vi "Get-file-names.vi"(8 "error in (no error)":errorcluster, 11 "Object ref in":T1) -> (0 "error out":errorcluster, 2 "Files list":string[][](array[string]), 3 "Object ref out":T1)   [LabVIEW 2013, in "SLMControl.lvlib" / "SC-Main.lvclass"]
uses:
  SC-Main.lvclass
  Object-reference.ctl
  UI/Control-names.ctl
  SC-Main.lvclass/SC-Main.ctl
  Read UI.vi
  Read Lasing files.vi
  Read Deposition files.vi
  UI/SC-UI.lvclass
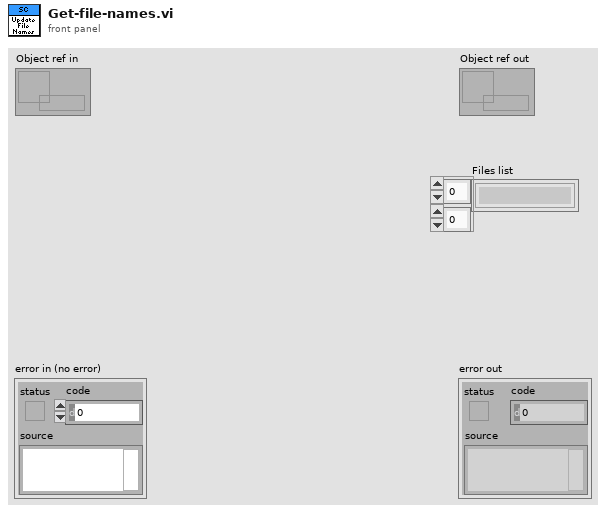
[diagram p1: front panel]
types:
  T1 = typedef "SLMControl.lvlib/SC-Main.lvclass/Object-reference.ctl" = refnum<data-value>
  T2 = typedef "SLMControl.lvlib/SC-UI.lvclass/Control-names.ctl" = enum16{"Com-in", "Com-out", "Help", "Status", "Load configuration", "Save configuration", "Load lasing files", "Load deposition files", "Clear", "Files", "Activate", "Execute", "Abort", "Options", "Current layer", "Current iteration", "Last elapsed time", "Deposition status", "Lasing job", "Status LEDs", "Exiting led", "Initialized led", "Files loaded led", "Activated led", "Executing led", "Deposition led", "Lasing job led", "Lasing led"}
  T3 = typedef "SLMControl.lvlib/SC-UI.lvclass/Panes-reference.ctl" = refnum<data-value>
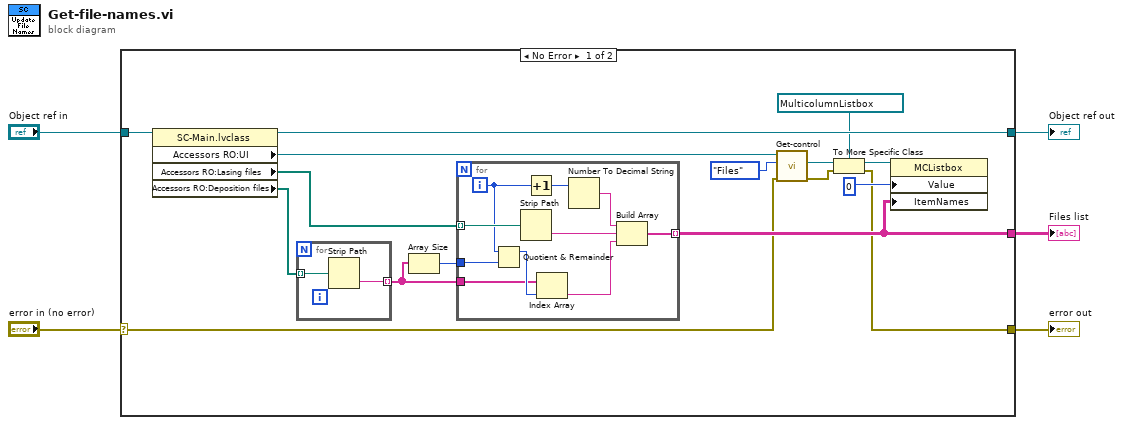
[diagram p0: block diagram]
diagram:
  n1 = case shown="No Error" "error in (no error)" {
    selector: "error in (no error)" -> [w8 w35]
    tunnel: [w6 w35] -> w4
    tunnel: [w20 w34] -> w2
    tunnel: "Object ref in" -> [w21 w34]
    tunnel: [w10 _] -> w1
    frame No Error {
      n2 = property class="SC-Main.lvclass"(reference=w21) -> (reference out=w20:T1, "Accessors RO:UI"=w15:T3, "Accessors RO:Lasing files"=w16:path[], "Accessors RO:Deposition files"=w19:path[])  [unwired: 1 in, 1 out]
      n3 = for {
        tunnel: w19 -> [w23] mode=indexing
        tunnel: [w22] -> w17 mode=indexing
        n4 = Strip Path(path=w23) -> (name=w22:string)  [unwired: 1 out]
      }
      n5 = Array Size(array=w17) -> (size(s)=w18:i32)
      n6 = for {
        tunnel: w16 -> [w33] mode=indexing
        tunnel: [w24] -> w10 mode=indexing
        tunnel: w17 -> [w26]
        tunnel: w18 -> [w29]
        i -> [w28]
        n7 = Quotient & Remainder(x=w28, y=w29) -> (x-y*floor(x/y)=w27:i32)  [unwired: 1 out]
        n8 = Strip Path(path=w33) -> (name=w30:string)  [unwired: 1 out]
        n9 = Increment(x=w28) -> (x+1=w32:i32)
        n10 = Index Array(array=w26, index=w27) -> (element=w25:string)
        n11 = Number To Decimal String(number=w32) -> (decimal integer string=w31:string)  [unwired: 1 in]
        n12 = Build Array(w31, w30, w25) -> (w24:string[])
      }
      n13 = call "Get-control.vi"("error in (no error)"=w8, "Control name"=Control-names."Files", "Panes in"=w15) -> ("error out"=w7:errorcluster, "Ctl Refnum"=w13:refnum<vi>)  [unwired: 6 in, 1 out]
      n14 = To More Specific Class(target class=refnum<vi> refnum ("Files"), reference=w13, error in=w7) -> (specific class reference=w12:refnum<vi>, error out=w6:errorcluster)
      n15 = property class="MCListbox"(reference=w12, "Value"=0, "ItemNames"=w10) -> ()  [unwired: 1 in, 2 out]
    }
    frame Error {
    }
  }
  "error out" <- w4
  "Object ref out" <- w2
  "Files list" <- w1
